vi "main.vi"(1 "Czy rysować kolor ?":bool, 2 "Liczba sąsiadów od środka":u32=1 min=1, 3 "Skalowanie":u32=1 min=1, 4 "Środek":u16[](array[numeric]), 5 "Wektor Bazowy 2":dbl[](array[numeric]), 6 "Wektor Bazowy 1":dbl[](array[numeric])) -> (0 "Wynik":picture)   [LabVIEW 2016]
panel:
  in  "Przybliżenie":sgl(slide)=0.1 min=0.1 max=10 step=0.1 scale=0.1..10.0
  in  "zatrzymaj symulacje":bool
  # "Rysowanie powyżej 5 sąsiadów może być bardzo\nCzasochłone i wymagające dla komputera"
  # "Nie"
  # "Tak"
  # "Wektory bazowe tworzące sieć\nNie dawać wektoró zerowych"
  # "Można nie rysować koloru\nw celu otrzymania bardziej\ndokładnego obrazu [konury są \ndobre do danego sąsiada\n(zależy od Liczbą sądiadów\nod środka), natomiast kolory\nsą takie same dla stref o tym\n\"samym promieniu\" od środka]"
  # "Ile jedna jednostka długości sieci \nreprezentuje pikseli na obrazku\nZaleca wartośc to przynajmniej 50"
  # "Środek sieci czyli pkt (0,0)\nOdnosi się to do pozycji na obrazie\n0 0 to lewy górny róg , a 900 900\nto prawy dolny róg\nZaleca się ustawić na około 450 450"
  # "Górne kontrolki są używane przed rysowaniem, dolne można zmienić w dowolnej chwili"
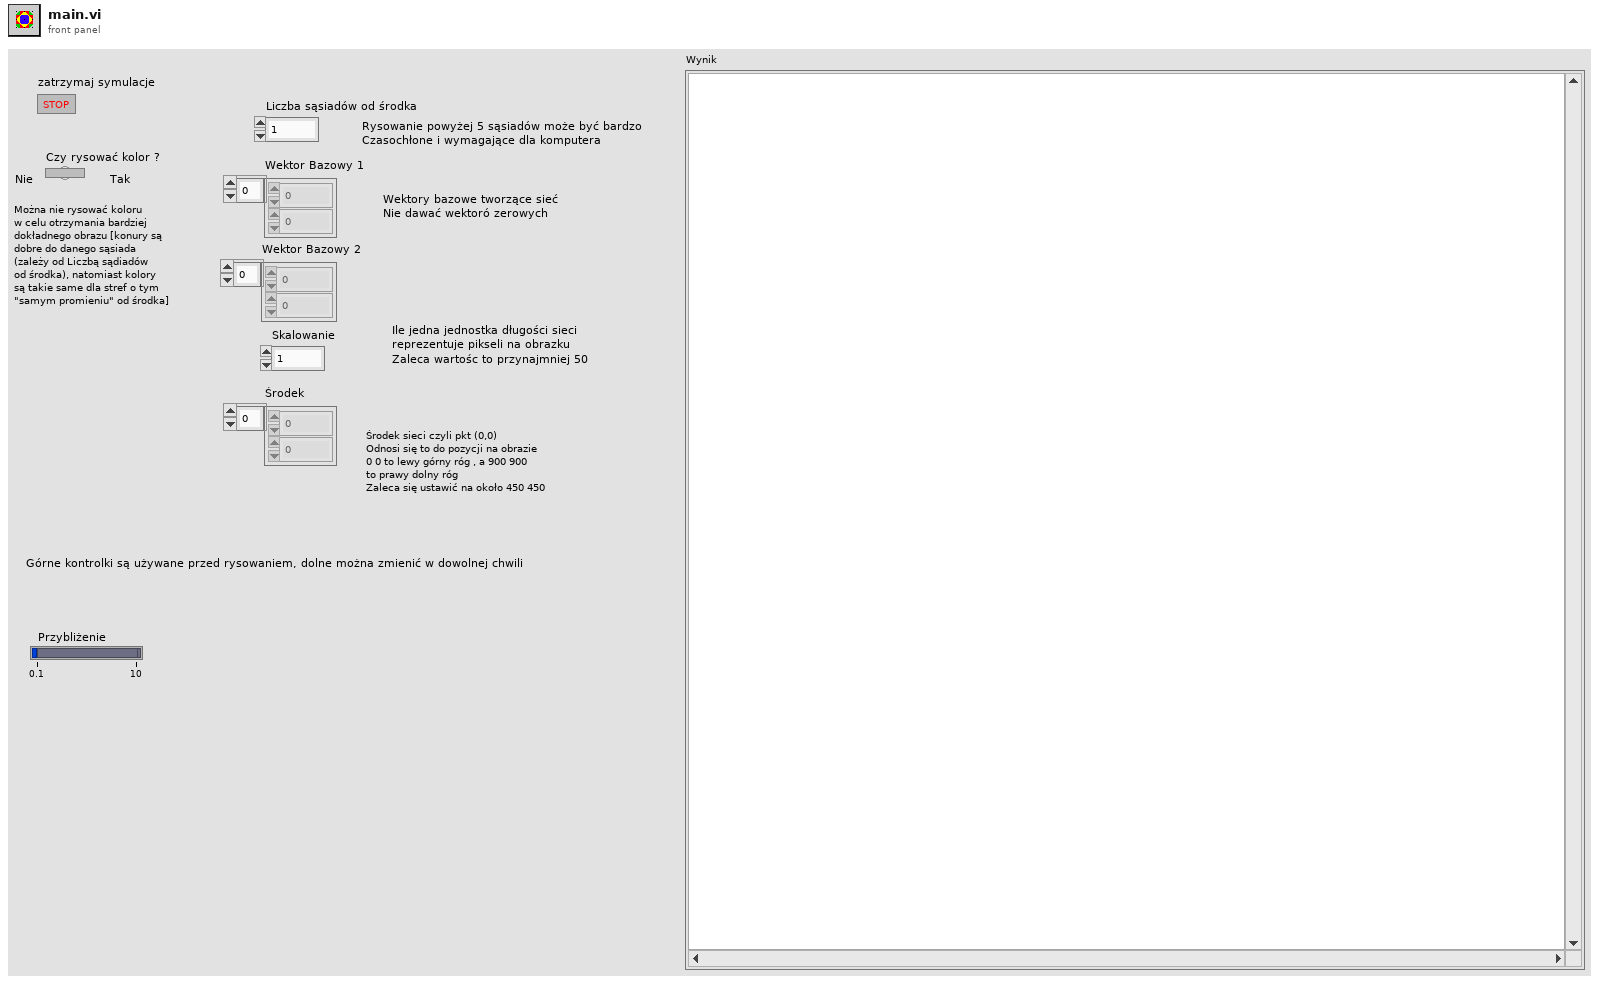
[diagram p1: front panel]
types:
  T1 = cluster{"Width":u16, "Style":enum32{"Solid", "Dash", "Dot", "DashDot", "DashDotDot"}}
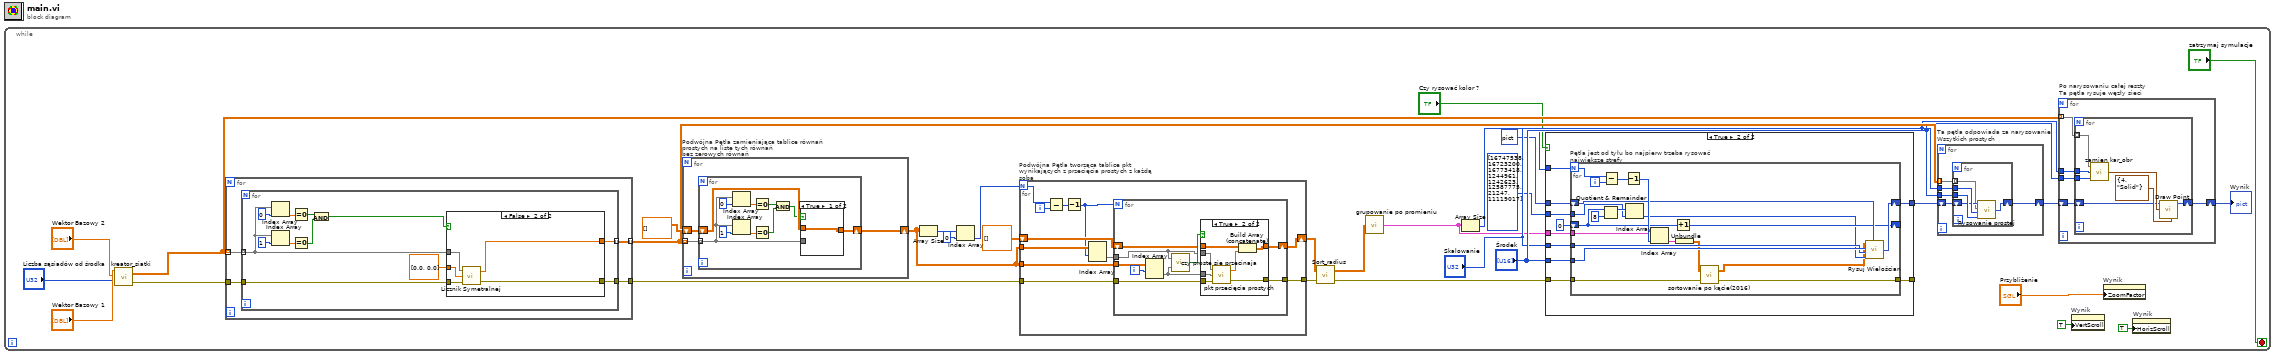
[diagram p0: block diagram]
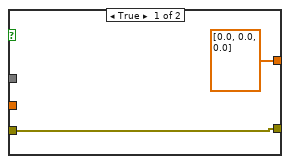
[diagram p4: hidden frame]
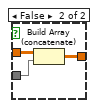
[diagram p5: hidden frame]
diagram:
  n1 = while {
    stop <- "zatrzymaj symulacje" stop-if-true
    n2 = call "kreator_siatki.vi"("Liczba Przejść"="Liczba sąsiadów od środka", "Wektor 2"="Wektor Bazowy 2", "Wektor 1"="Wektor Bazowy 1") -> ("error out"=w27:errorcluster, "Tablica pkt"=w26:dbl[][][])  [unwired: 1 in]
    n3 = for {
      tunnel: w26 -> [w118] mode=indexing
      tunnel: w27 -> [w117]
      tunnel: [w116] -> w23 mode=indexing
      tunnel: [w115] -> w21
      n4 = for {
        tunnel: w118 -> [w120] mode=indexing
        tunnel: w117 -> [w123]
        tunnel: [w121] -> w116 mode=indexing
        tunnel: [w119] -> w115
        n5 = Index Array(array=w120, index=0) -> (element=w128:dbl)
        n6 = Index Array(array=w120, index=1) -> (element=w127:dbl)
        n7 = Equal To 0?(x=w128) -> (x = 0?=w126:bool)
        n8 = Equal To 0?(x=w127) -> (x = 0?=w125:bool)
        n9 = And(x=w126, y=w125) -> (x .and. y?=w124:bool)
        n10 = case shown="False" w124 {
          tunnel: w123 -> [w131 w137]
          tunnel: dbl[] [0.0, 0.0] ("Array 2") -> [_ w136]
          tunnel: [dbl[] [0.0, 0.0, 0.0] ("appended array") w135] -> w121
          tunnel: w120 -> [_ w134]
          tunnel: [w131 w133] -> w119
          frame True {
          }
          frame False {
            n11 = call "Licznik Symetralnej.vi"("error in"=w137, "Punkt 2"=w136, "Punkt 1"=w134) -> ("error out"=w133:errorcluster, "równanie prostej"=w135:dbl[])
          }
        }
      }
    }
    n12 = for "Podwójna Pętla zamieniająca tablice równań prostych na liste tych równań\nbez zerowych równań" {
      shift-right: [w139] -> w20
      shift-left: dbl[][] [] ("element") -> [w140]
      tunnel: w23 -> [w138] mode=indexing
      n13 = for {
        shift-right: [w149] -> w139
        shift-left: w140 -> [w150]
        tunnel: w138 -> [w148] mode=indexing
        n14 = Index Array(array=w148, index=0) -> (element=w145:dbl)
        n15 = Index Array(array=w148, index=1) -> (element=w144:dbl)
        n16 = Equal To 0?(x=w145) -> (x = 0?=w143:bool)
        n17 = Equal To 0?(x=w144) -> (x = 0?=w142:bool)
        n18 = And(x=w143, y=w142) -> (x .and. y?=w141:bool)
        n19 = case shown="True" w141 {
          tunnel: w150 -> [w151 w154]
          tunnel: w148 -> [_ w153]
          tunnel: [w151 w152] -> w149
          frame True {
          }
          frame False {
            n20 = Build Array (concatenate)(w154, w153) -> (w152:dbl[][])
          }
        }
      }
    }
    n21 = Array Size(array=w20) -> (size(s)=w19:i32[])
    n22 = Index Array(array=w19, index=0) -> (element=w17:i32)
    n23 = for "Podwójna Pętla tworząca tablice pkt wynikających z przecięcia prostych z każdą sobą" {
      N: w17 -> [w73]
      tunnel: w20 -> [w67]
      tunnel: w20 -> [w74]
      tunnel: w21 -> [w71]
      tunnel: [w70] -> w16
      shift-right: [w68] -> w15
      shift-left: dbl[][] [] ("element") -> [w69]
      i -> [w72]
      n24 = Subtract(x=w73, y=w72) -> (x-y=w66:i32)
      n25 = Decrement(x=w66) -> (x-1=w64:i32)
      n26 = Index Array(array=w67, index (row)=w64) -> (element=w65:dbl[])  [unwired: 1 in]
      n27 = for {
        N: w64 -> [_]
        tunnel: w74 -> [w77]
        tunnel: w65 -> [w82]
        tunnel: w71 -> [w81]
        tunnel: [w80] -> w70
        shift-right: [w78] -> w68
        shift-left: w69 -> [w79]
        i -> [w76]
        n28 = Index Array(array=w77, index (row)=w76) -> (element=w75:dbl[])  [unwired: 1 in]
        n29 = call "czy proste sie przecinaja.vi"("Równanie Prostej 2"=w75, "Równanie Prostej 1"=w82) -> ("czy się przecinają ?"=w83:bool)
        n30 = case shown="True" w83 {
          tunnel: w82 -> [_ w92]
          tunnel: w75 -> [_ w91]
          tunnel: w81 -> [w85 w90]
          tunnel: [w85 w89] -> w80
          tunnel: w79 -> [w84 w87]
          tunnel: [w84 w86] -> w78
          frame False {
          }
          frame True {
            n31 = call "pkt przecięcia prostych.vi"("error in"=w90, "Równanie Prostej 2"=w91, "Równanie Prostej 1"=w92) -> ("error out"=w89:errorcluster, "Punkt Przecięcia"=w88:dbl[])
            n32 = Build Array (concatenate)(w87, w88) -> (w86:dbl[][])
          }
        }
      }
    }
    n33 = call "Sort_radius.vi"("error in"=w16, "unsorted array"=w15) -> ("error out"=w14:errorcluster, "Array"=w6:dbl[][])
    n34 = call "grupowanie po promieniu.vi"("Posortowana Tablica\nPo promieniu"=w6) -> ("Grupy pkt \nO tych samych\nPromieniach"=w5:cluster{dbl[][]}[])
    n35 = Array Size(array=w5) -> (size(s)=w4:i32)
    n36 = case shown="True" "Czy rysować kolor ?" {
      tunnel: w14 -> [w32 w41]
      tunnel: "Środek" -> [_ w40]
      tunnel: "Skalowanie" -> [_ w38]
      tunnel: u32[] [16747538, 16723200, 16773418, 1244961, 1242623, 12587775, 21247, 11119017] -> [_ w39]
      tunnel: picture data[5B] ("picture") -> [w33 w42]
      tunnel: [w33 w36] -> w9
      tunnel: w5 -> [_ w43]
      tunnel: [w32 w37] -> _
      tunnel: w4 -> [_ w34]
      frame False {
      }
      frame True {
        n37 = for "Pętla jest od tyłu bo najpierw trzeba rysować największe strefy" {
          N: w34 -> [w63]
          tunnel: w43 -> [w59]
          shift-right: [w52] -> w36
          shift-left: w42 -> [w54]
          tunnel: w41 -> [w58]
          tunnel: w40 -> [w57]
          tunnel: w39 -> [w56]
          tunnel: w38 -> [w55]
          tunnel: [w53] -> w37
          shift-right: [w51] -> _
          shift-left: 0 -> [w44]
          i -> [w62]
          n38 = Quotient & Remainder(x=w44, y=u32 8) -> (x-y*floor(x/y)=w48:u32)  [unwired: 1 out]
          n39 = Subtract(x=w63, y=w62) -> (x-y=w61:i32)
          n40 = Decrement(x=w61) -> (x-1=w60:i32)
          n41 = Index Array(array=w56, index=w48) -> (element=w46:u32)
          n42 = Index Array(array=w59, index=w60) -> (element=w50:cluster{dbl[][]})
          n43 = Increment(x=w44) -> (x+1=w51:i32)
          n44 = Unbundle(w50) -> (w47:dbl[][])
          n45 = call "sortowanie po kącie(2016).vi"("error in (no error)"=w58, "unsorted array"=w47) -> ("error out"=w53:errorcluster, "sorted array"=w45:dbl[][])
          n46 = call "Rysuj Wielościan.vi"("tablica punktów"=w45, "Środek"=w57, "przeskalowanie"=w55, "color"=w46, "przed rysunkiem"=w54) -> ("po rysunku"=w52:picture)
        }
      }
    }
    n47 = for "Ta pętla odpowiada za narysowanie\nWszytkich prostych" {
      tunnel: w23 -> [w109] mode=indexing
      tunnel: "Skalowanie" -> [w108]
      tunnel: "Środek" -> [w107]
      shift-right: [w105] -> w25
      shift-left: w9 -> [w106]
      n48 = for {
        tunnel: w109 -> [w110] mode=indexing
        tunnel: w108 -> [w114]
        tunnel: w107 -> [w113]
        shift-right: [w111] -> w105
        shift-left: w106 -> [w112]
        n49 = call "Rysowanie prostej.vi"("Środek"=w113, "Skalowanie"=w114, "Równanie prostej"=w110, "picture"=w112) -> ("new picture"=w111:picture)
      }
    }
    n50 = for "Po narysowaniu całej reszty\nTa pętla rysuje węzły sieci" {
      tunnel: w26 -> [w97] mode=indexing
      tunnel: "Środek" -> [w96]
      tunnel: "Skalowanie" -> [w95]
      shift-right: [w93] -> w24
      shift-left: w25 -> [w94]
      n51 = for {
        tunnel: w97 -> [w104] mode=indexing
        tunnel: w96 -> [w103]
        tunnel: w95 -> [w102]
        shift-right: [w98] -> w93
        shift-left: w94 -> [w99]
        n52 = call "zamien kar_obr.vi"("Środek"=w103, "Skalowanie"=w102, "Pkt"=w104) -> ("pkt we wsp obrazu"=w100:cluster{i16, i16})
        n53 = call <vilib>:"Draw Point.vi"("picture"=w99, "point(x,y)"=w100, "pen"=T1 {"Width"=4, "Style"=enum."Solid"}) -> ("new picture"=w98:picture)  [unwired: 6 in]
      }
    }
    "Wynik" <- w24
    n54 = property on="Wynik" class="Pict"("VertScroll"=TRUE ("Vertical Scrollbar Visible")) -> ()  [unwired: 2 in, 2 out]
    n55 = property on="Wynik" class="Pict"("ZoomFactor"="Przybliżenie") -> ()  [unwired: 2 in, 2 out]
    n56 = property on="Wynik" class="Pict"("HorizScroll"=TRUE ("Horizontal Scrollbar Visible")) -> ()  [unwired: 2 in, 2 out]
  }
